vi "Max Search.vi"() -> ()   [LabVIEW 2024]
panel:
  out "Max":dbl
  out "Iterations":i32
  in  "Number of Iterations":i32
  out "Random Number":dbl
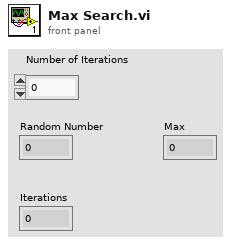
[diagram p1: front panel]
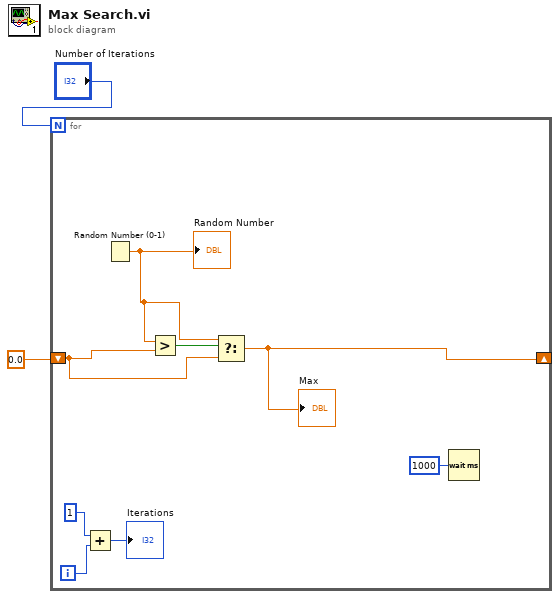
[diagram p0: block diagram]
diagram:
  n1 = for {
    N: "Number of Iterations" -> [_]
    shift-right: [w3] -> _
    shift-left: 0.0 -> [w5]
    i -> [w8]
    n2 = Add(x=1, y=w8) -> (x+y=→"Iterations":i32)
    n3 = Random Number (0-1)() -> (number: 0 to 1=w6:dbl)
    "Random Number" <- w6
    n4 = Greater?(x=w6, y=w5) -> (0:w4:bool)
    n5 = Select(t=w6, s=w4, f=w5) -> (s? t:f=w3:dbl)
    "Max" <- w3
    n6 = Wait (ms)(milliseconds to wait=u32 1000) -> ()  [unwired: 1 out]
  }
